vi "PS Get MEasure Params.vi"(10 "Ring Text":string, 11 "PS Measure Type 2":refnum<vi>) -> ()   [LabVIEW 2020]
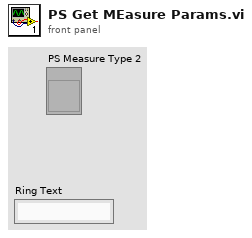
[diagram p1: front panel]
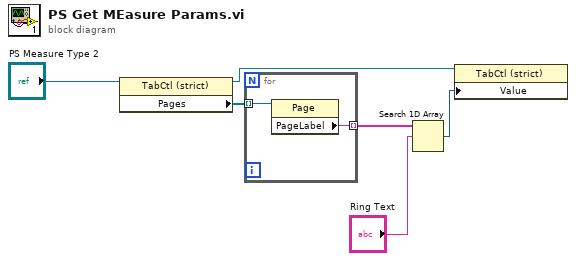
[diagram p0: block diagram]
diagram:
  n1 = property class="TabCtl (strict)"(reference="PS Measure Type 2") -> (reference out=w2:refnum<vi>, "Pages"=w5:refnum<vi>[])  [unwired: 1 in, 1 out]
  n2 = for {
    tunnel: w5 -> [w8] mode=indexing
    tunnel: [w7] -> w4 mode=indexing
    n3 = property class="Page"(reference=w8) -> ("PageLabel"=w7:string)  [unwired: 1 in, 2 out]
  }
  n4 = Search 1D Array(1D array=w4, element="Ring Text") -> (index of element=w1:i32)  [unwired: 1 in]
  n5 = property class="TabCtl (strict)"(reference=w2, "Value"=w1) -> ()  [unwired: 1 in, 2 out]
